vi "Read Process Variable and Setpoint.vi"(8 "error in (no error)":errorcluster, 11 "PID Loop in":refnum<class "PID Loop.lvclass">) -> (0 "error out":errorcluster, 1 "process variable":dbl, 2 "setpoint":dbl, 3 "PID Loop out":refnum<class "PID Loop.lvclass">)   [LabVIEW 2024, in "PID Loop.lvlib" / "PID Loop.lvclass"]
uses:
  PID Loop.lvclass
  PID Loop.lvclass/PID Loop.ctl
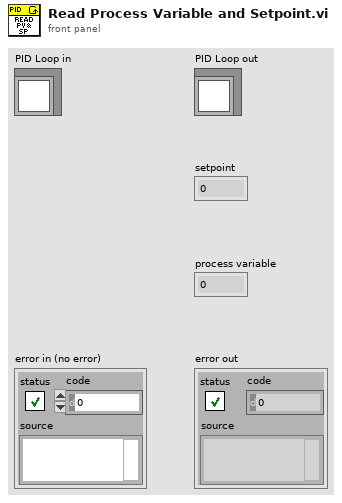
[diagram p1: front panel]
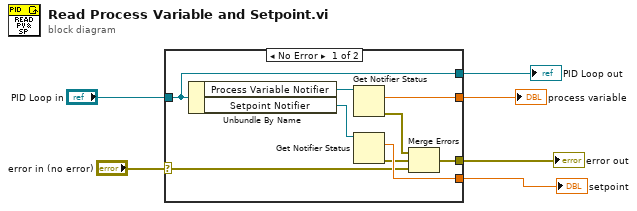
[diagram p0: block diagram]
diagram:
  n1 = case shown="No Error" "error in (no error)" {
    selector: "error in (no error)" -> [w7 w17]
    tunnel: [w8 w17] -> w5
    tunnel: [w15 w16] -> w3
    tunnel: "PID Loop in" -> [w15 w16]
    tunnel: [w12 _] -> w2
    tunnel: [w11 _] -> w1
    frame No Error {
      n2 = Unbundle By Name(w15) -> ("Process Variable Notifier"=w14:refnum<notifier>, "Setpoint Notifier"=w13:refnum<notifier>)
      n3 = Get Notifier Status(notifier=w14) -> (current notification=w12:dbl, error out=w10:errorcluster)  [unwired: 1 in, 3 out]
      n4 = Get Notifier Status(notifier=w13) -> (current notification=w11:dbl, error out=w9:errorcluster)  [unwired: 1 in, 3 out]
      n5 = Merge Errors(w10, w9, w7) -> (w8:errorcluster)
    }
    frame Error {
    }
  }
  "error out" <- w5
  "PID Loop out" <- w3
  "process variable" <- w2
  "setpoint" <- w1
